vi "Log Error.vi"(5 "Current state":T1, 7 "Car Position Slider":T2 scale=0.0..4.0, 8 "error in":errorcluster, 9 "Source":string, 10 "Code":i32, 11 "Error Log Refnum In":refnum<file>) -> (0 "error out":errorcluster, 3 "Error Log Refnum Out":refnum<file>)   [LabVIEW 2017]
uses:
  controls/Position Slider.ctl
  controls/Current State.ctl
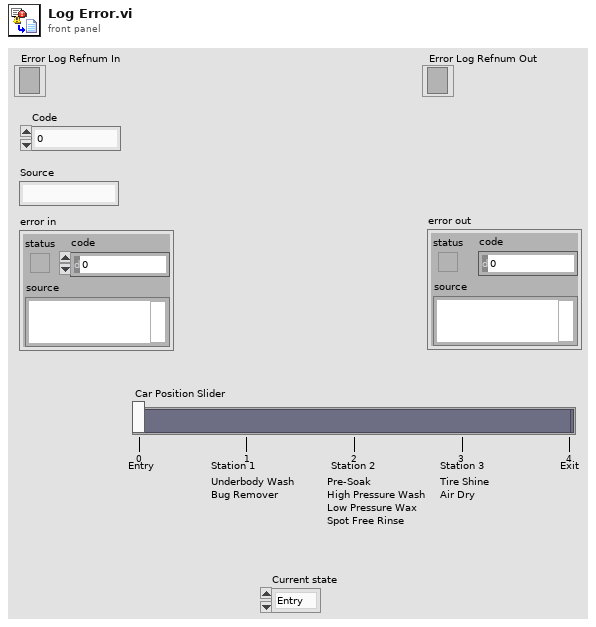
[diagram p1: front panel]
types:
  T1 = typedef "Current State.ctl" = enum16{"Entry", "Under Body Wash", "Bug Remover", "Pre-Soak", "High Pressure Wash", "Low Pressure Wax", "Spot Free Rinse", "Tire Shine Foam", "Air Dry", "Exit"}
  T2 = typedef "Position Slider.ctl" = i32
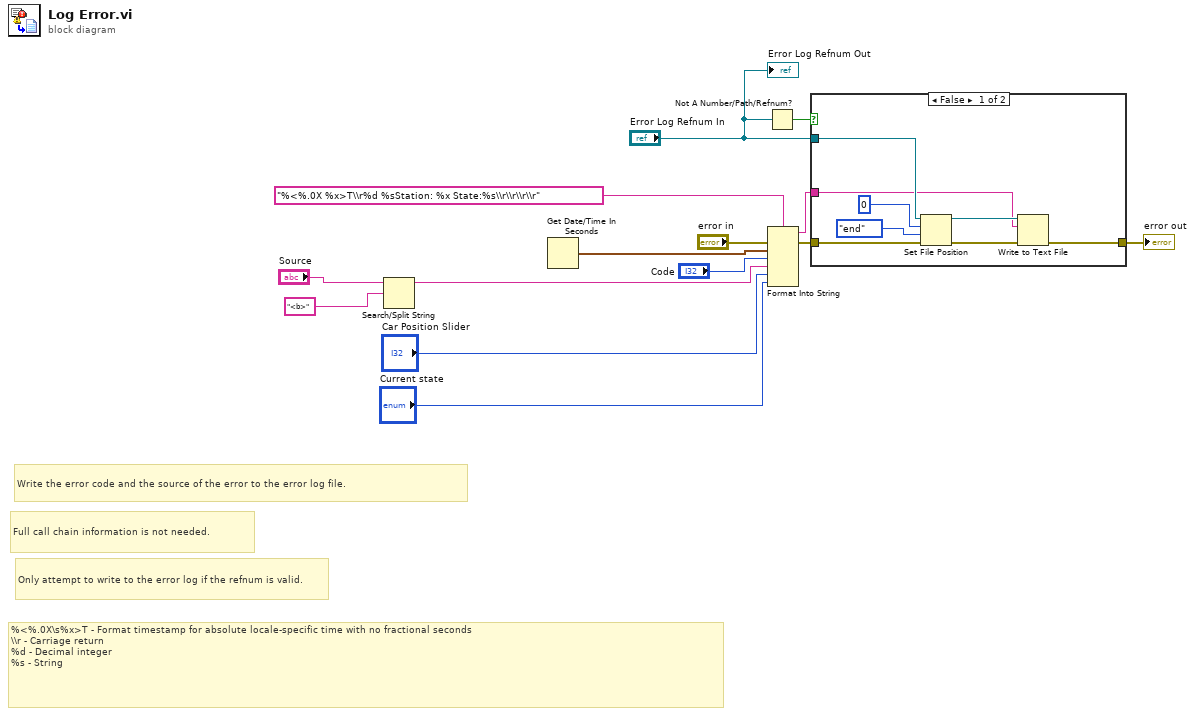
[diagram p0: block diagram]
diagram:
  # "Full call chain information is not needed."
  # "Only attempt to write to the error log if the refnum is valid."
  # "%<%.0X\\s%x>T - Format timestamp for absolute locale-specific time with no fractional seconds\n\\\\r - Carriage return\n%d - Decimal integer\n%s - String"
  # "Write the error code and the source of the error to the error log file."
  n1 = Search/Split String(string="Source", search string/char (-)="<b>") -> (substring before match=w5:string)  [unwired: 1 in, 2 out]
  n2 = Get Date/Time In Seconds() -> (seconds since 1Jan1904=w3:timestamp)
  n3 = Not A Number/Path/Refnum?(number/path/refnum="Error Log Refnum In") -> (NaN/Path/Refnum?=w9:bool)
  n4 = Format Into String(format string="%<%.0X %x>T\\r%d %sStation: %x State:%s\\r\\r\\r\\r", error in="error in", w3, "Code", w5, "Car Position Slider", "Current state") -> (resulting string=w13:string, error out=w14:errorcluster)  [unwired: 1 in]
  n5 = case shown="False" w9 {
    tunnel: w14 -> [w18 w23]
    tunnel: w13 -> [w17 _]
    tunnel: [w22 w23] -> w11
    tunnel: "Error Log Refnum In" -> [w20 _]
    frame False {
      n6 = Set File Position(offset (in bytes) (0)=i64 0, refnum=w20, from (0:start)=enum16{"start", "end", "current"}."end", error in=w18) -> (refnum out=w19:refnum<file>, error out=w21:errorcluster)
      n7 = Write to Text File(file (use dialog)=w19, text=w17, error in=w21) -> (error out=w22:errorcluster)  [unwired: 1 in, 2 out]
    }
    frame True {
    }
  }
  "error out" <- w11
  "Error Log Refnum Out" <- "Error Log Refnum In"
